vi "getAll.vi"(8 "error in (no error)":errorcluster, 11 "VNA":refnum<class "VNA.lvclass">) -> (0 "error out":errorcluster, 2 "getAll":variant, 3 "VNA out":refnum<class "VNA.lvclass">)   [LabVIEW 2016, in "VNA.lvclass"]
uses:
  VNA.lvclass
  <userlib>/LevyLab/Levylab Instruments/Instrument Types/VNA/Instrument.VNA.lvclass
  P:/users1/Dengyu/Agilent 87XX Series/Agilent 87XX Series.lvlib
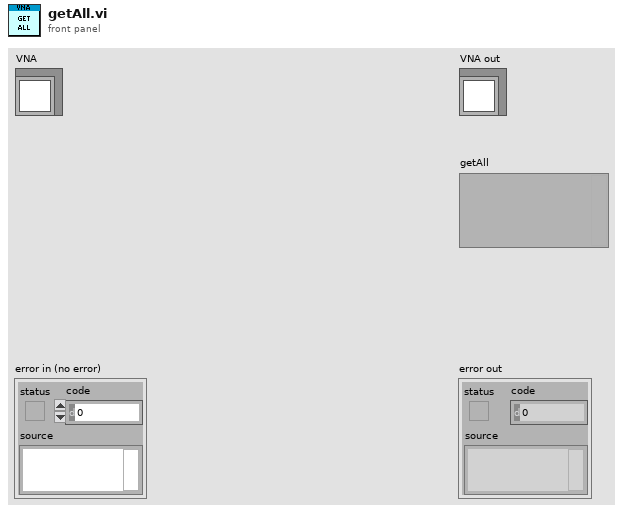
[diagram p1: front panel]
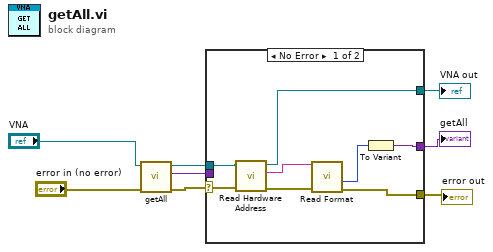
[diagram p0: block diagram]
diagram:
  n1 = call-parent "getAll.vi"("error in (no error)"="error in (no error)", "Instrument in"="VNA") -> ("error out"=w6:errorcluster, "getAll"=w1:variant, "Instrument out"=w4:refnum<class "VNA.lvclass">)  [unwired: 7 in]
  n2 = case shown="No Error" w6 {
    selector: w6 -> [w15 w19]
    tunnel: [w16 w19] -> w5
    tunnel: w4 -> [w13 w17]
    tunnel: [w10 w18] -> w3
    tunnel: [w11 w17] -> w2
    tunnel: w1 -> [_ w18]
    frame No Error {
      n3 = call-dynamic "Read Hardware Address.vi"("error in (no error)"=w15, "Instrument in"=w13) -> ("error out"=w14:errorcluster, "Hardware Address"=w12:string, "Instrument out"=w11:refnum<class "VNA.lvclass">)  [unwired: 7 in]
      n4 = call "Read Format.vi"("error in (no error)"=w14, "VISA resource name"=w12) -> ("error out"=w16:errorcluster, "format"=w9:i32)  [unwired: 7 in, 1 out]
      n5 = To Variant(anything=w9) -> (Variant=w10:variant)
    }
    frame Error {
    }
  }
  "error out" <- w5
  "VNA out" <- w2
  "getAll" <- w3
